vi "tvac_gui.vi"() -> ()   [LabVIEW 2017]
uses:
  <vilib>/httpClient/ClientHandle.ctl
  msg7171_linux.llb/send single message.vi
  <vilib>/httpClient/POSTBuffer.vi
  <vilib>/httpClient/LabVIEWHTTPClient.lvlib
panel:
  in  "Local Debug":bool
  out "Index Values":u32[](array[numeric])
  in  "NumberTCs":i32=120
  in  "Tab Control":enum32{"TCs"}(tab)
  in  "Graphing Selection":u16(ring) items=["User Selection", "Graph All Thermocouples", "Clear Graph"]
  in  "Time Scale":u16(ring) items=["Minutes", "Hours", "Seconds"]
  out "Waveform Chart":waveform(dbl)[](graph)
  out "Thermocouples":T1(array[cluster])
  in  "exit":bool
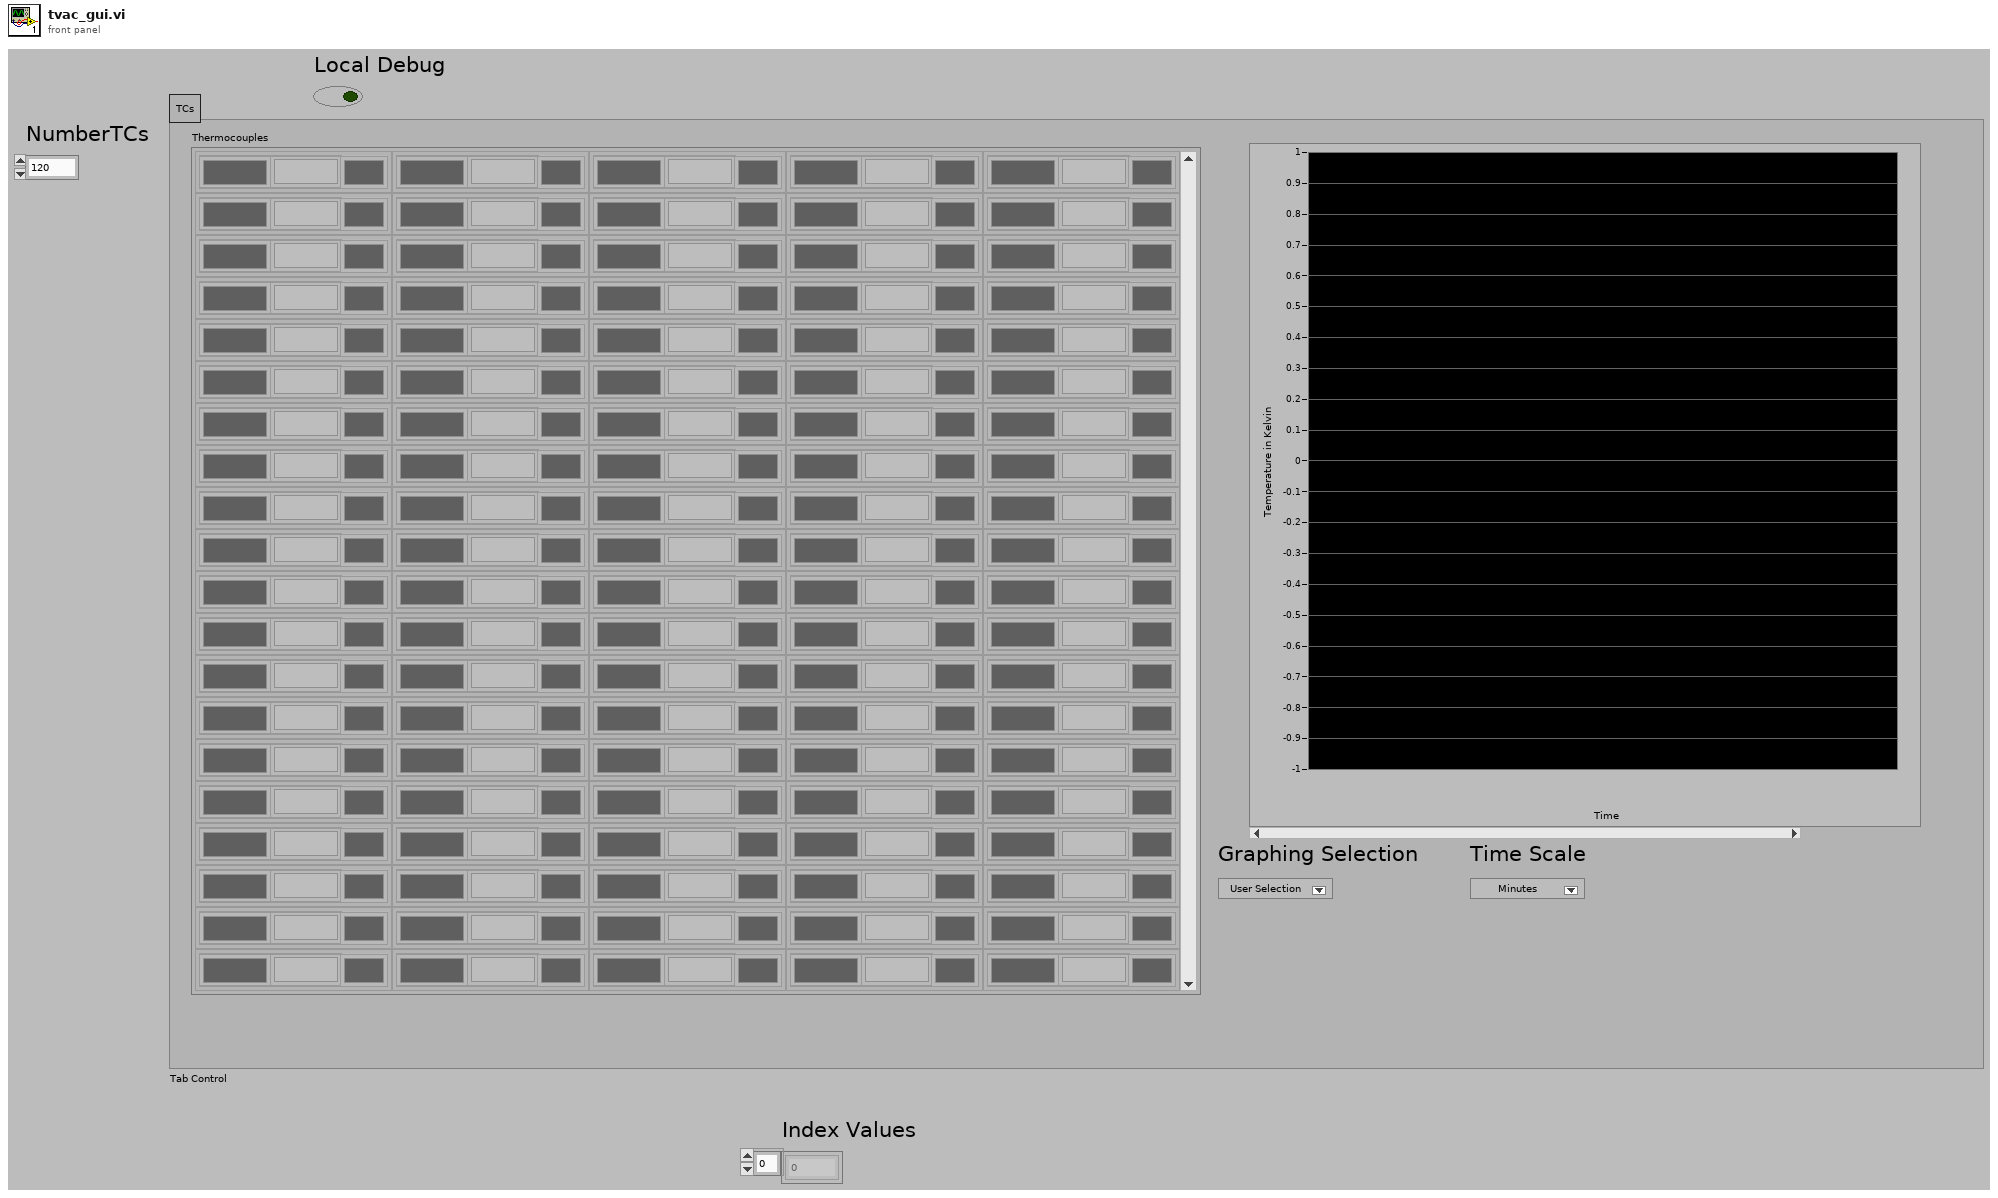
[diagram p1: front panel]
types:
  T1 = cluster{"TC Label":string, "Alarm Status":string, "Alarm Color":u32, "Temperature":string, "PlotColor":u32, "Graph On/Off":u32}[][]
  T2 = typedef "LabVIEWHTTPClient.lvlib/ClientHandle.ctl" = refnum<k1>
  T3 = cluster{"go":bool, "Http session":T2, "URL prefex":string}
  T4 = typedef "LVPoint32TypeDef.ctl" = cluster{"Horizontal":i32, "Vertical":i32}
  T5 = typedef "LVPositionTypeDef.ctl" = cluster{"Left":i32, "Top":i32}
  T6 = cluster{"TC Label":string, "Alarm Status":string, "Alarm Color":u32, "Temperature":string, "PlotColor":u32, "Graph On/Off":u32}
  T7 = typedef "LVRangeTypeDef.ctl" = cluster{"Minimum":dbl, "Maximum":dbl, "Increment":dbl, "Minor Increment":dbl, "Start":dbl}
  T8 = cluster{"time":string, "TCs":cluster{"thermocouple":i32, "time":dbl, "temp":dbl, "working":bool, "alarm":i32}[]}
  T9 = cluster{"thermocouple":i32, "time":dbl, "temp":dbl, "working":bool, "alarm":i32}[]
  T10 = cluster{"thermocouple":i32, "time":dbl, "temp":dbl, "working":bool, "alarm":i32}
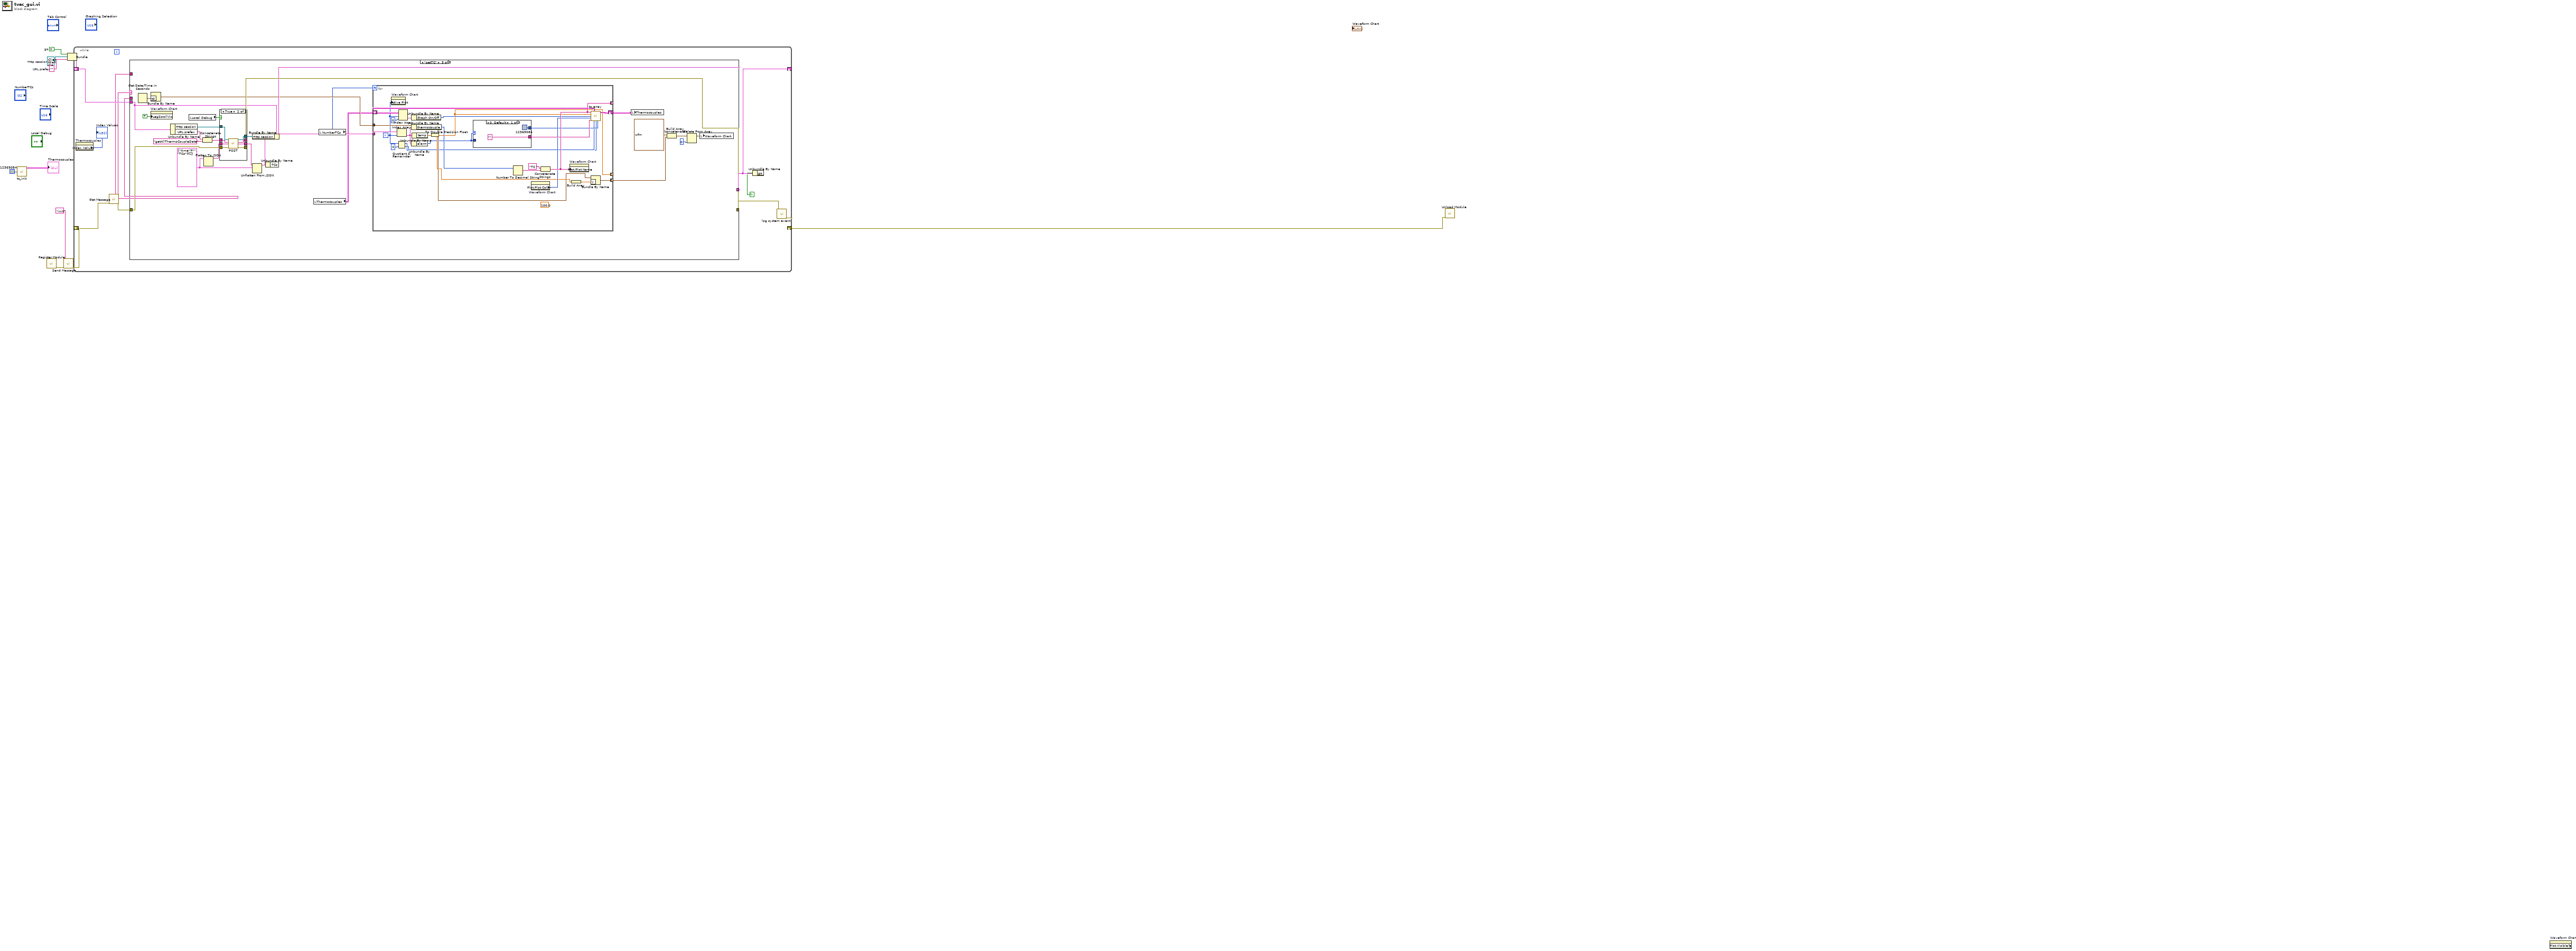
[diagram p0: block diagram]
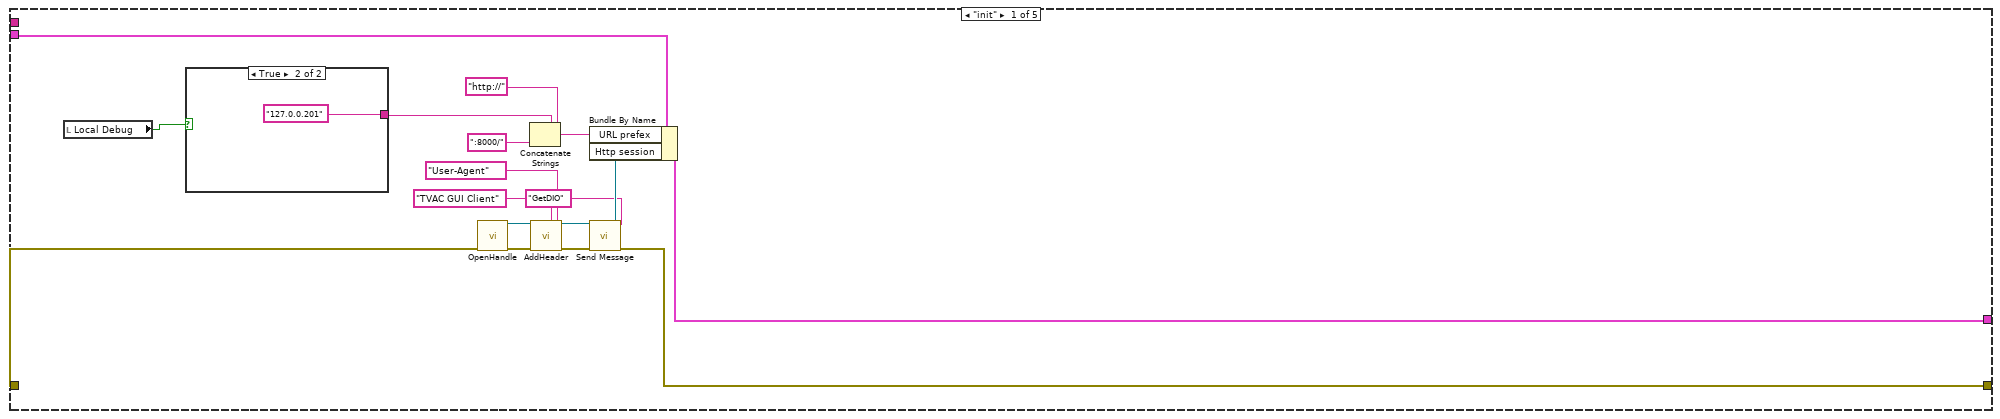
[diagram p2: hidden frame]
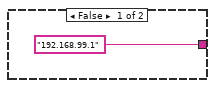
[diagram p3: hidden frame]
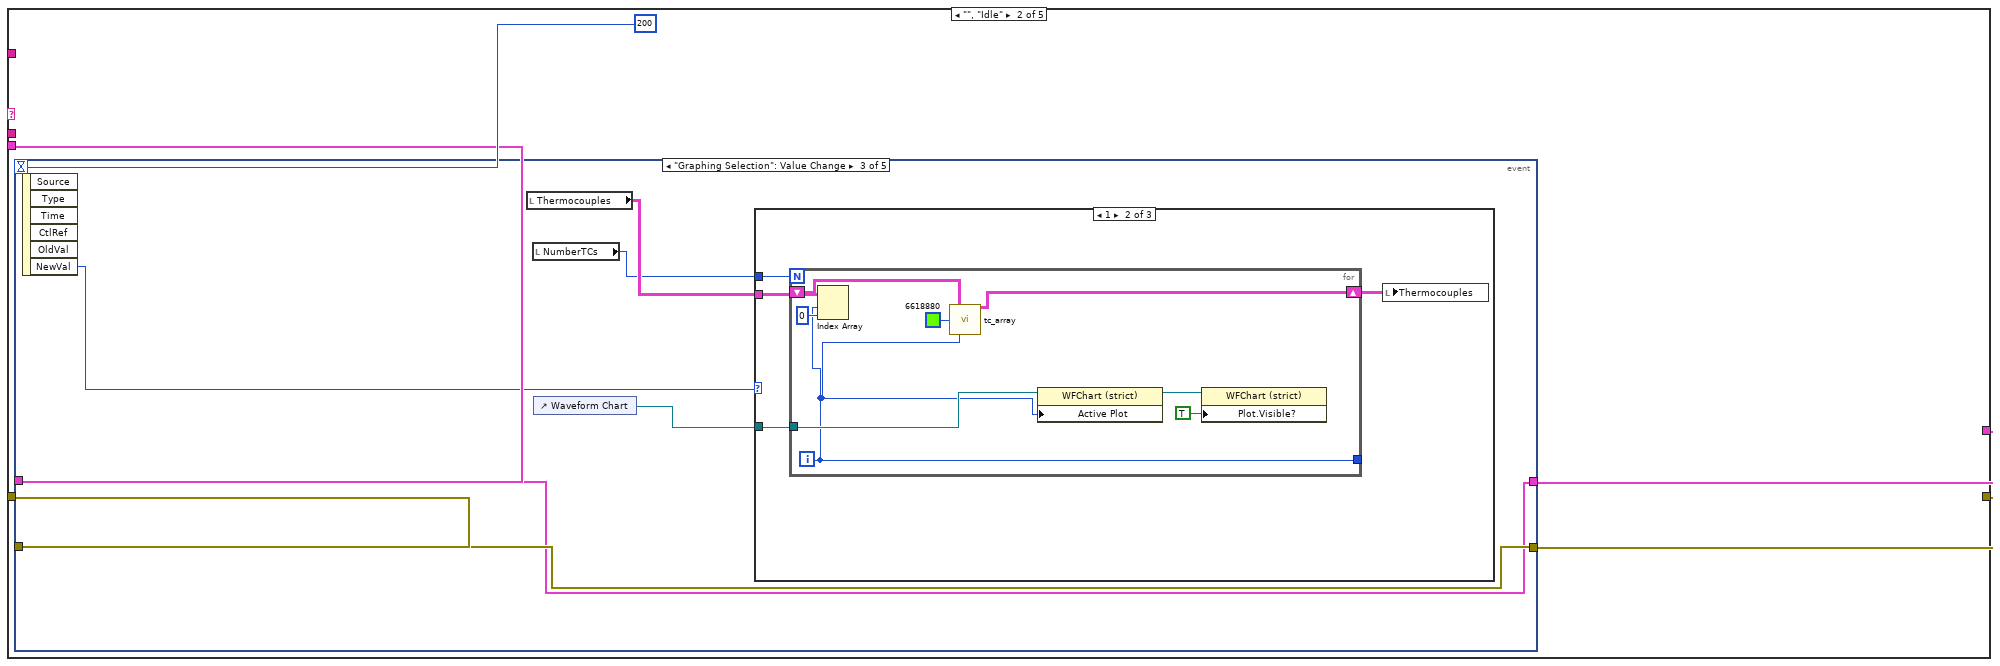
[diagram p4: hidden frame]
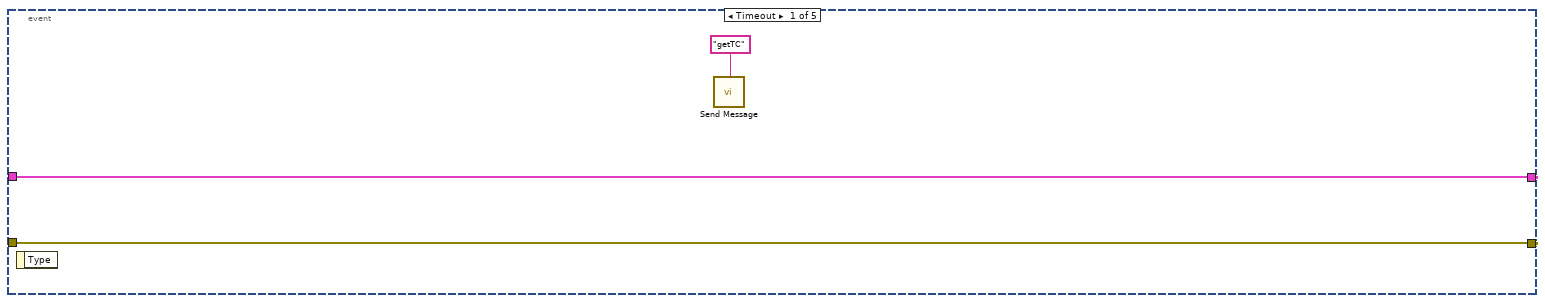
[diagram p5: hidden frame]
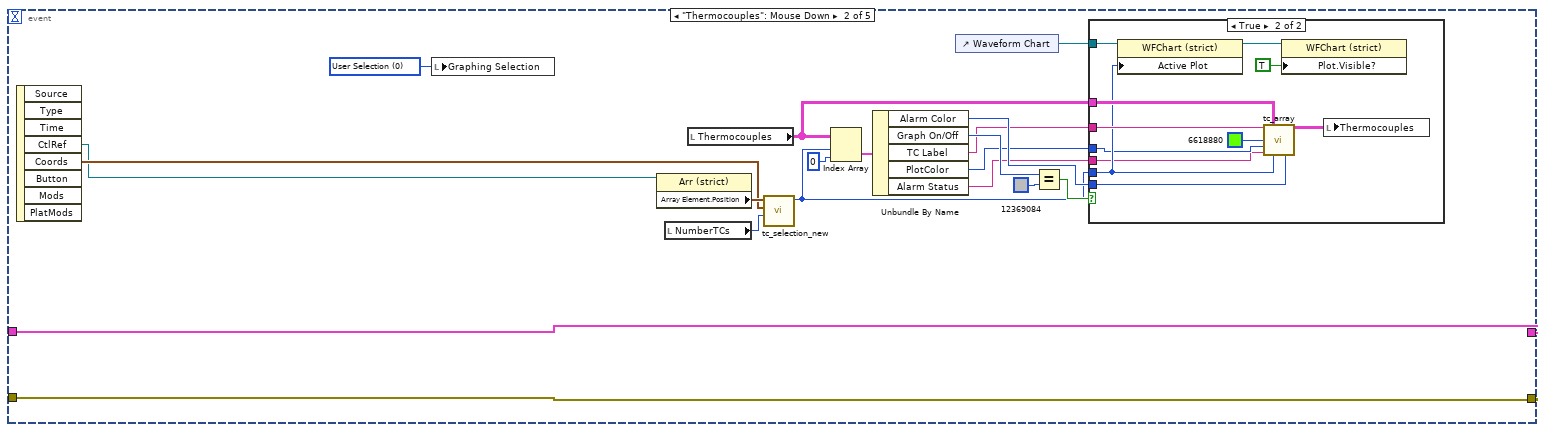
[diagram p6: hidden frame]
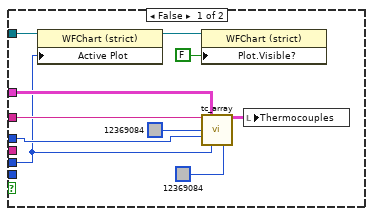
[diagram p7: hidden frame]
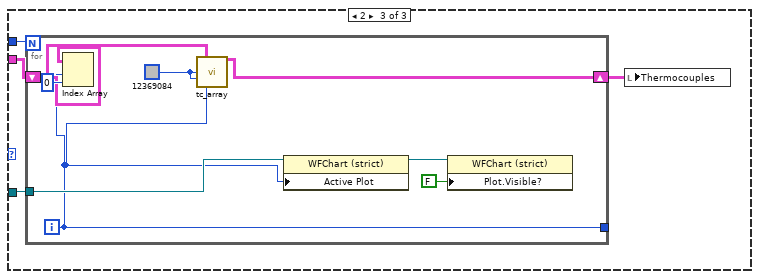
[diagram p9: hidden frame]
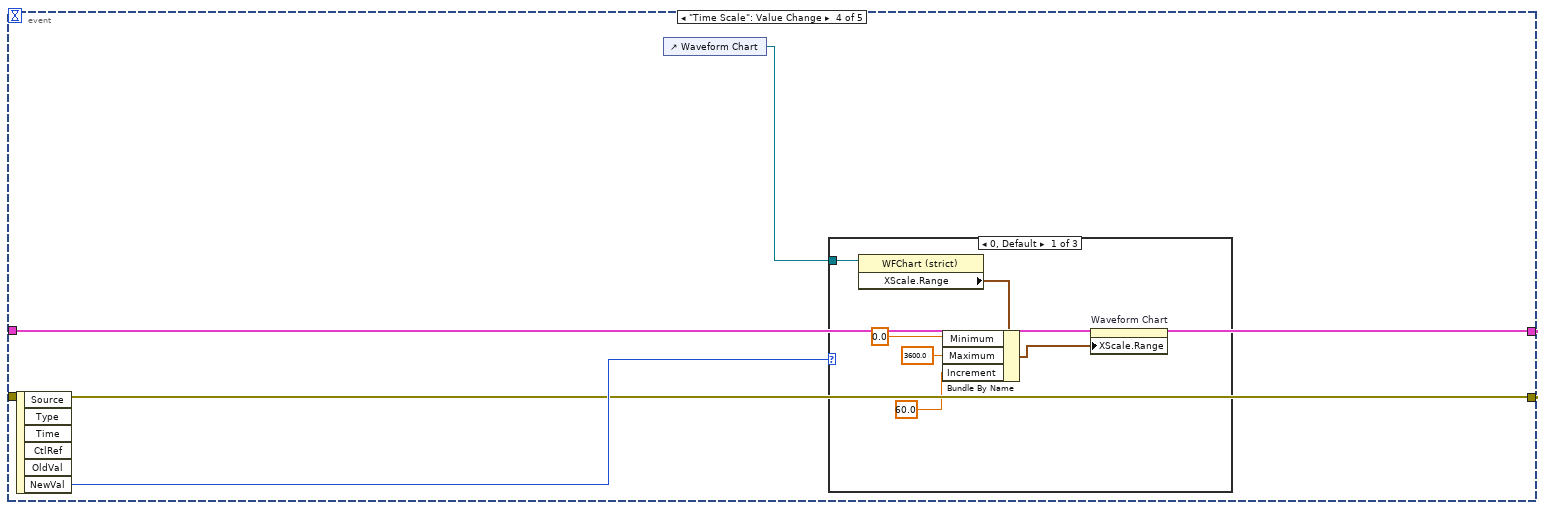
[diagram p10: hidden frame]
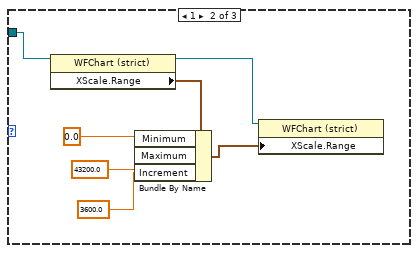
[diagram p11: hidden frame]
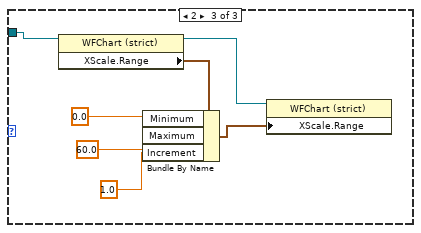
[diagram p12: hidden frame]
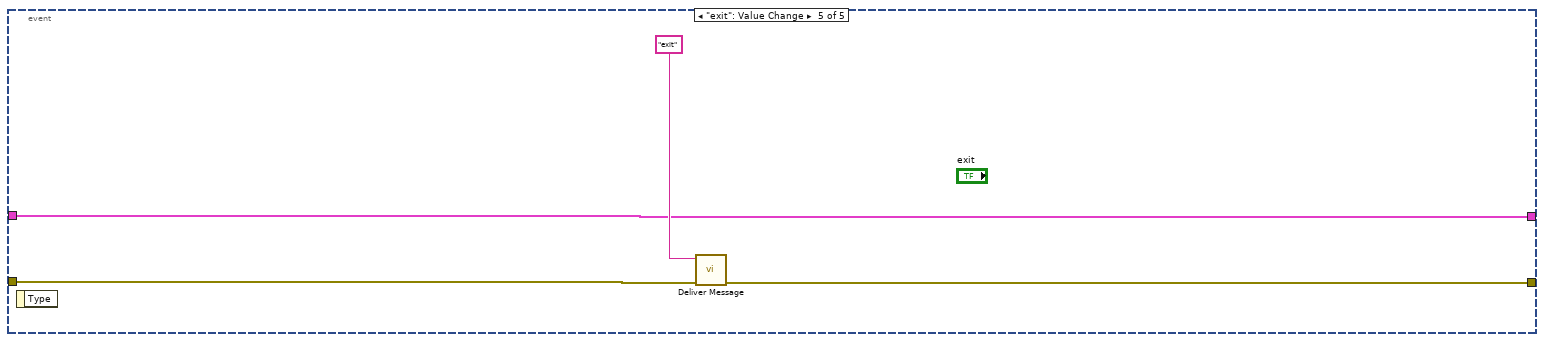
[diagram p13: hidden frame]
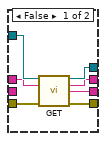
[diagram p14: hidden frame]
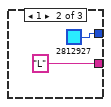
[diagram p15: hidden frame]
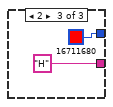
[diagram p16: hidden frame]
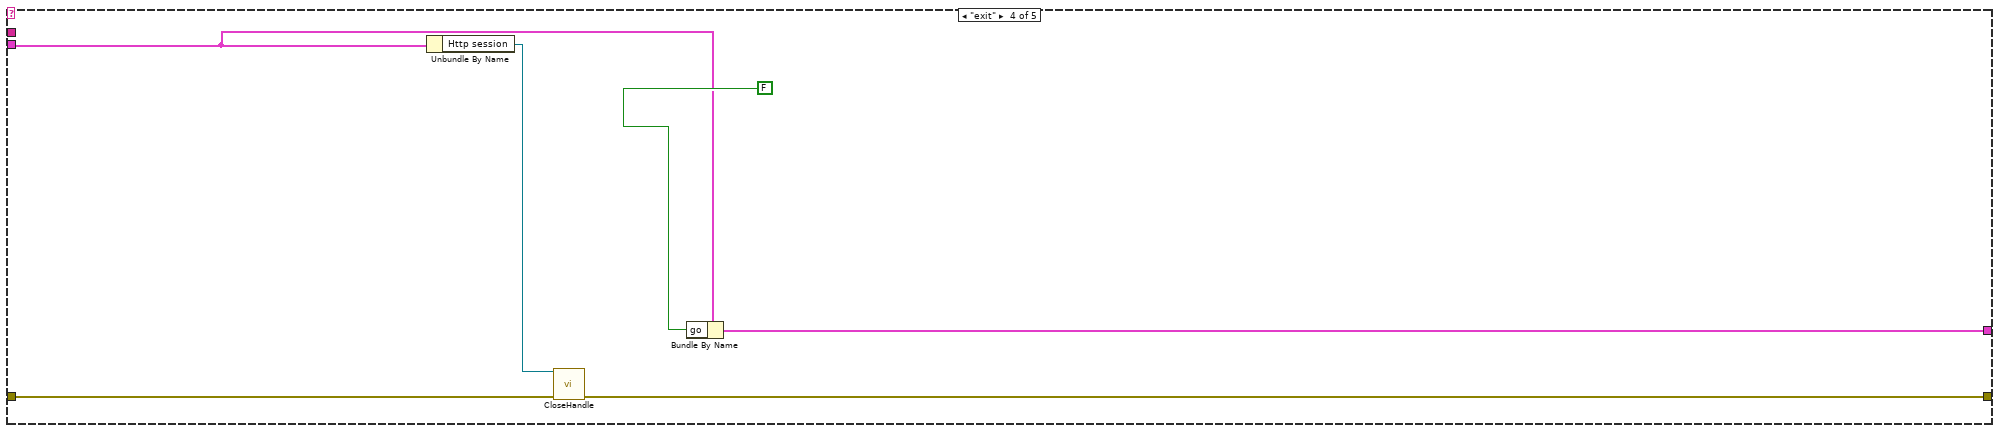
[diagram p17: hidden frame]
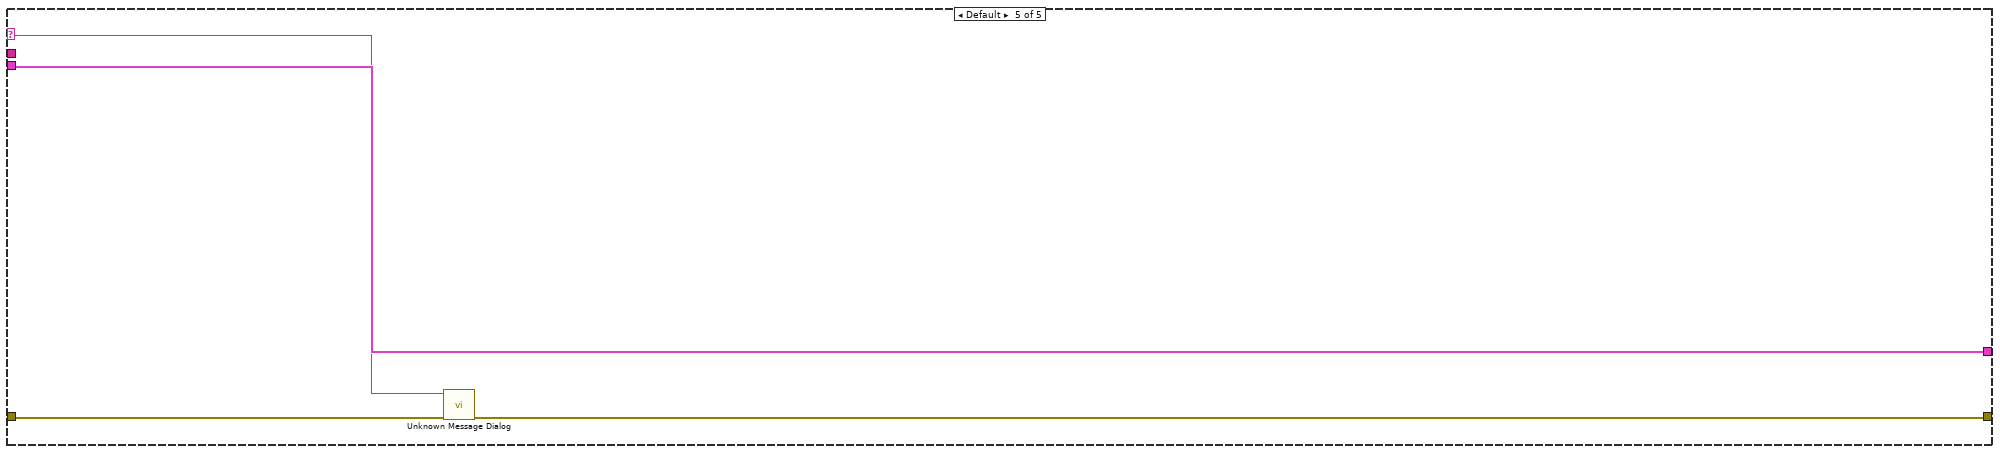
[diagram p18: hidden frame]
diagram:
  w6 = ""  # URL prefex
  w7 = T2 refnum  # Http session
  w8 = TRUE  # go
  n1 = call "tc_init.vi"("Graph ON/OFF"=u32 12369084) -> ("output array"=→"Thermocouples":T1)  [unwired: 14 in]
  n2 = call "Register Module.vi"() -> ("error out"=w4:errorcluster)  [unwired: 10 in, 1 out]
  n3 = call-poly "Send Message.vi"("error in (no error)"=w4, "event"="init") -> ("error out"=w3:errorcluster)  [unwired: 9 in]
  n4 = Bundle("go"=w8, "Http session"=w7, "URL prefex"=w6) -> (w10:T3)  [unwired: 1 in]
  n5 = while {
    shift-left: w10 -> [w18]
    shift-right: [w16] -> _
    shift-right: [w15] -> w9
    shift-left: w3 -> [w21]
    stop <- w12 continue-if-true
    n6 = property on="Thermocouples" class="Arr (strict)"() -> ("Index Values"=→"Index Values":u32[])  [unwired: 2 in, 2 out]
    n7 = call "Get Message.vi"("error in (no error)"=w21) -> ("error out"=w19:errorcluster, "event buffer"=w20:string, "event"=w17:string, "source"=w13:string)  [unwired: 7 in]
    n8 = case shown="\"getTC\"" w17 {
      selector: w17 -> [_ _ _ _ w224]
      tunnel: [w29 w41 w169 w222 w226] -> w16
      tunnel: w18 -> [w37 w40 w167 w217 w226]
      tunnel: w20 -> [_ _ _ _ _]
      tunnel: w19 -> [w32 w42 w171 w220 w225]
      tunnel: [w25 w44 w170 w219 w223] -> w14
      tunnel: w13 -> [_ _ _ _ _]
      frame "init" {
        n9 = local read "Local Debug"() -> (w22:bool)
        n10 = case shown="True" w22 {
          tunnel: ["192.168.99.1" ("Address") "127.0.0.201" ("Address")] -> w23
          frame False {
          }
          frame True {
          }
        }
        n11 = call <vilib>:"OpenHandle.vi"("error in (no error)"=w32) -> ("client handle out"=w33:T2, "error out"=w36:errorcluster)  [unwired: 13 in]
        n12 = Concatenate Strings("http://" ("url"), w23, ":8000/" ("url")) -> (w28:string)
        n13 = call <vilib>:"AddHeader.vi"("client handle"=w33, "header"="User-Agent", "value"="TVAC GUI Client", "error in (no error)"=w36) -> ("client handle out"=w27:T2, "error out"=w26:errorcluster)  [unwired: 10 in]
        n14 = Bundle By Name(cluster=w37, "URL prefex"=w28, "Http session"=w27) -> (w29:T3)
        n15 = call-poly "Send Message.vi"("error in (no error)"=w26, "event"="GetDIO") -> ("error out"=w25:errorcluster)  [unwired: 9 in]
      }
      frame "", "Idle" {
        n16 = event shown="[2] \"Graphing Selection\": Value Change" {
          selector: _ -> [_ _ _ _ _]
          dyn-events: _ -> [_ _ _ _ _]
          timeout: 200 ("milliseconds to wait") -> [_ _ _ _ _]
          tunnel: w42 -> [w46 w66 w89 w119 w145]
          tunnel: [w46 w66 w89 w119 w144] -> w44
          tunnel: [w47 w65 w88 w120 w142] -> w41
          tunnel: w40 -> [w47 w65 w88 w120 w142]
          event Timeout {
            n17 = event-data() -> ()  [unwired: 1 in, 1 out]
            n18 = call-poly "Send Message.vi"("event"="getTC") -> ()  [unwired: 10 in, 1 out]
          }
          event "Thermocouples": Mouse Down {
            w48 = u16 0 items=["User Selection", "Graph All Thermocouples", "Clear Graph"] ("Graphing Selection")
            n19 = event-data() -> ("CtlRef"=w62:refnum<vi>, "Coords"=w63:T4)  [unwired: 1 in, 6 out]
            n20 = local write "Graphing Selection"(w48) -> ()
            n21 = property class="Arr (strict)"(reference=w62) -> ("Array Element.Position"=w64:T5)  [unwired: 1 in, 2 out]
            n22 = local read "NumberTCs"() -> (w54:i32)
            n23 = local read "Thermocouples"() -> (w56:T1)
            n24 = call "tc_selection_new.vi"("Numeric 2"=w54, "Coords"=w63, "Position"=w64) -> ("Numeric"=w50:i32)  [unwired: 8 in]
            n25 = Index Array(array=w56, index (row)=w50, index (col)=0 ("disabled index (col)")) -> (element=w59:T6)
            n26 = Unbundle By Name(w59) -> ("Alarm Color"=w55:u32, "Graph On/Off"=w53:u32, "TC Label"=w52:string, "PlotColor"=w51:u32, "Alarm Status"=w49:string)
            n27 = control-ref of="Waveform Chart"() -> (w57:refnum<vi>)
            n28 = Equal?(x=w53, y=u32 12369084) -> (x = y?=w58:bool)
            n29 = case shown="True" w58 {
              tunnel: w50 -> [w68 w80]
              tunnel: w57 -> [w74 w85]
              tunnel: w56 -> [w70 w82]
              tunnel: w55 -> [_ w77]
              tunnel: w52 -> [w72 w84]
              tunnel: w51 -> [w69 w79]
              tunnel: w49 -> [_ w78]
              frame False {
                n30 = property on="Property Node" class="WFChart (strict)"(reference=w74, "Active Plot"=w68) -> (reference out=w75:refnum<vi>)  [unwired: 1 in, 1 out]
                n31 = property class="WFChart (strict)"(reference=w75, "Plot.Visible?"=FALSE ("Plot.Visible")) -> ()  [unwired: 1 in, 2 out]
                n32 = call "tc_array.vi"("TC Label"=w72, "output array 2"=w70, "Graph ON/OFF"=u32 12369084, "Plot Color"=w69, "index (row)"=w68, "AlarmColor"=u32 12369084) -> ("output array"=w71:T1)  [unwired: 9 in]
                n33 = local write "Thermocouples"(w71) -> ()
              }
              frame True {
                n34 = property class="WFChart (strict)"(reference=w85, "Active Plot"=w80) -> (reference out=w86:refnum<vi>)  [unwired: 1 in, 1 out]
                n35 = call "tc_array.vi"("TC Label"=w84, "output array 2"=w82, "Graph ON/OFF"=u32 6618880, "Plot Color"=w79, "Alarm String"=w78, "index (row)"=w80, "AlarmColor"=w77) -> ("output array"=w81:T1)  [unwired: 8 in]
                n36 = property class="WFChart (strict)"(reference=w86, "Plot.Visible?"=TRUE ("Plot.Visible")) -> ()  [unwired: 1 in, 2 out]
                n37 = local write "Thermocouples"(w81) -> ()
              }
            }
          }
          event "Graphing Selection": Value Change {
            n38 = event-data() -> ("NewVal"=w90:u16)  [unwired: 1 in, 5 out]
            n39 = local read "Thermocouples"() -> (w93:T1)
            n40 = local read "NumberTCs"() -> (w91:i32)
            n41 = control-ref of="Waveform Chart"() -> (w92:refnum<vi>)
            n42 = case shown="1" w90 {
              tunnel: w93 -> [_ w97 w108]
              tunnel: w92 -> [_ w96 w107]
              tunnel: w91 -> [_ w95 w109]
              frame 0, Default {
              }
              frame 1 {
                n43 = for {
                  N: w95 -> [_]
                  tunnel: w96 -> [w102]
                  tunnel: [w101] -> _
                  shift-right: [w99] -> w94
                  shift-left: w97 -> [w100]
                  i -> [w101]
                  n44 = Index Array(array=w100, index (row)=w101, index (col)=0 ("disabled index (col)")) -> ()  [unwired: 1 out]
                  n45 = call "tc_array.vi"("output array 2"=w100, "Graph ON/OFF"=u32 6618880, "index (row)"=w101) -> ("output array"=w99:T1)  [unwired: 12 in]
                  n46 = property class="WFChart (strict)"(reference=w102, "Active Plot"=w101) -> (reference out=w104:refnum<vi>)  [unwired: 1 in, 1 out]
                  n47 = property class="WFChart (strict)"(reference=w104, "Plot.Visible?"=TRUE ("Plot.Visible")) -> ()  [unwired: 1 in, 2 out]
                }
                n48 = local write "Thermocouples"(w94) -> ()
              }
              frame 2 {
                n49 = for {
                  N: w109 -> [_]
                  tunnel: w107 -> [w114]
                  tunnel: [w112] -> _
                  shift-right: [w110] -> w106
                  shift-left: w108 -> [w113]
                  i -> [w112]
                  w111 = u32 12369084
                  n50 = Index Array(array=w113, index (row)=w112, index (col)=0 ("disabled index (col)")) -> ()  [unwired: 1 out]
                  n51 = call "tc_array.vi"("output array 2"=w113, "Graph ON/OFF"=w111, "Plot Color"=w111, "index (row)"=w112) -> ("output array"=w110:T1)  [unwired: 11 in]
                  n52 = property class="WFChart (strict)"(reference=w114, "Active Plot"=w112) -> (reference out=w116:refnum<vi>)  [unwired: 1 in, 1 out]
                  n53 = property class="WFChart (strict)"(reference=w116, "Plot.Visible?"=FALSE ("Plot.Visible")) -> ()  [unwired: 1 in, 2 out]
                }
                n54 = local write "Thermocouples"(w106) -> ()
              }
            }
          }
          event "Time Scale": Value Change {
            n55 = event-data() -> ("NewVal"=w121:u16)  [unwired: 1 in, 5 out]
            n56 = control-ref of="Waveform Chart"() -> (w118:refnum<vi>)
            n57 = case shown="0, Default" w121 {
              tunnel: w118 -> [w125 w129 w136]
              frame 0, Default {
                n58 = property on="Property Node" class="WFChart (strict)"(reference=w125) -> ("XScale.Range"=w127:T7)  [unwired: 1 in, 2 out]
                n59 = Bundle By Name(cluster=w127, "Minimum"=0.0, "Maximum"=3600.0, "Increment"=60.0) -> (w126:T7)
                n60 = property on="Waveform Chart" class="WFChart (strict)"("XScale.Range"=w126) -> ()  [unwired: 2 in, 2 out]
              }
              frame 1 {
                n61 = property on="Property Node" class="WFChart (strict)"(reference=w129) -> (reference out=w128:refnum<vi>, "XScale.Range"=w134:T7)  [unwired: 1 in, 1 out]
                n62 = Bundle By Name(cluster=w134, "Minimum"=0.0, "Maximum"=43200.0, "Increment"=3600.0) -> (w130:T7)
                n63 = property on="Property Node" class="WFChart (strict)"(reference=w128, "XScale.Range"=w130) -> ()  [unwired: 1 in, 2 out]
              }
              frame 2 {
                n64 = property on="Property Node" class="WFChart (strict)"(reference=w136) -> (reference out=w135:refnum<vi>, "XScale.Range"=w141:T7)  [unwired: 1 in, 1 out]
                n65 = Bundle By Name(cluster=w141, "Minimum"=0.0, "Maximum"=60.0, "Increment"=1.0) -> (w137:T7)
                n66 = property on="Property Node" class="WFChart (strict)"(reference=w135, "XScale.Range"=w137) -> ()  [unwired: 1 in, 2 out]
              }
            }
          }
          event "exit": Value Change {
            n67 = event-data() -> ()  [unwired: 1 in, 1 out]
            n68 = call "Deliver Message.vi"("error in (no error)"=w145, "event"="exit") -> ("error out"=w144:errorcluster)  [unwired: 9 in]
          }
        }
      }
      frame "getTC" {
        w148 = T8 {"time"="", "TCs"=[]} ("Cluster")
        n69 = Get Date/Time In Seconds() -> (seconds since 1Jan1904=w157:timestamp)
        n70 = Bundle By Name("t0"=w157) -> (w156:waveform(dbl))  [unwired: 1 in]
        n71 = property on="Waveform Chart" class="WFChart (strict)"("LegScrollVis"=TRUE ("Legend:Scrollbar Visible")) -> ()  [unwired: 2 in, 2 out]
        n72 = Unbundle By Name(w167) -> ("Http session"=w166:T2, "URL prefex"=w164:string)
        n73 = local read "Local Debug"() -> (w146:bool)
        n74 = Concatenate Strings(w164, "getAllThermoCoupleData" ("url")) -> (w165:string)
        n75 = Flatten To JSON(anything=w148) -> (JSON string=w147:string)  [unwired: 2 in, 1 out]
        n76 = case shown="True" w146 {
          tunnel: w171 -> [w178 w179]
          tunnel: [w177 w180] -> w170
          tunnel: [w176 w181] -> w168
          tunnel: w166 -> [w175 w184]
          tunnel: w165 -> [w174 w185]
          tunnel: [w173 w182] -> w162
          tunnel: [w172 w183] -> _
          tunnel: w147 -> [_ w186]
          frame False {
            n77 = call <vilib>:"GET.vi"("client handle"=w175, "url"=w174, "error in (no error)"=w178) -> ("client handle out"=w176:T2, "headers"=w172:string, "body"=w173:string, "error out"=w177:errorcluster)  [unwired: 9 in]
          }
          frame True {
            n78 = call-poly <vilib>:"POST.vi"("client handle"=w184, "url"=w185, "buffer"=w186, "error in (no error)"=w179) -> ("client handle out"=w181:T2, "headers"=w183:string, "body"=w182:string, "error out"=w180:errorcluster)  [unwired: 8 in]
          }
        }
        n79 = Bundle By Name(cluster=w167, "Http session"=w168) -> (w169:T3)
        n80 = Unflatten From JSON(JSON string=w162, type and defaults=w148) -> (value=w161:T8)  [unwired: 5 in, 1 out]
        n81 = Unbundle By Name(w161) -> ("TCs"=w160:T9)
        n82 = local read "Thermocouples"() -> (w152:T1)
        n83 = local read "NumberTCs"() -> (w149:i32)
        n84 = for {
          N: w149 -> [_]
          tunnel: w160 -> [w210]
          tunnel: w156 -> [w208]
          tunnel: [w209] -> w155 mode=indexing
          tunnel: [w192] -> _ mode=indexing
          tunnel: [w198] -> _ mode=indexing
          shift-right: [w199] -> w153
          shift-left: w152 -> [w197]
          i -> [w189]
          (unwired) 100.0 ("x")
          n85 = property on="Waveform Chart" class="WFChart (strict)"("Active Plot"=w189) -> ()  [unwired: 2 in, 2 out]
          n86 = Quotient & Remainder(x=w189, y=4) -> (x-y*floor(x/y)=w187:i32, floor(x/y)=w188:i32)
          n87 = Index Array(array=w210, index=w189) -> (element=w202:T10)
          n88 = Index Array(array=w197, index (row)=w189, index (col)=0 ("disabled index (col)")) -> (element=w201:T6)
          n89 = Unbundle By Name(w201) -> ("Graph On/Off"=w194:u32)
          n90 = Unbundle By Name(w202) -> ("thermocouple"=w206:i32)
          n91 = Unbundle By Name(w202) -> ("alarm"=w191:i32)
          n92 = Unbundle By Name(w202) -> ("temp"=w204:dbl)
          n93 = To Double Precision Float(number=w204) -> (double precision float=w192:dbl)
          n94 = case shown="0, Default" w191 {
            tunnel: ["" "L" "H"] -> w196
            tunnel: w191 -> [_ _ _]
            tunnel: [u32 12369084 u32 2812927 u32 16711680] -> w193
            frame 0, Default {
            }
            frame 1 {
            }
            frame 2 {
            }
          }
          n95 = Number To Decimal String(number=w206) -> (decimal integer string=w207:string)  [unwired: 1 in]
          n96 = property on="Waveform Chart" class="WFChart (strict)"() -> ("Plot.Plot Color"=w195:u32)  [unwired: 2 in, 2 out]
          n97 = Concatenate Strings("TC " ("string"), w207) -> (w198:string)
          n98 = property on="Waveform Chart" class="WFChart (strict)"("Plot.Plot Name"=w198) -> ()  [unwired: 2 in, 2 out]
          n99 = Build Array(w192) -> (w203:dbl[])
          n100 = call "tc_array.vi"("TC Label"=w198, "output array 2"=w197, "Temperature"=w192, "Graph ON/OFF"=w194, "Plot Color"=w195, "Alarm String"=w196, "index (row)"=w188, "index (col)"=w187, "AlarmColor"=w193) -> ("output array"=w199:T1)  [unwired: 6 in]
          n101 = Bundle By Name(cluster=w208, "Y"=w203) -> (w209:waveform(dbl))
        }
        n102 = local write "Thermocouples"(w153) -> ()
        n103 = Build Array (concatenate)(waveform(dbl) {"t0"=timestamp(0 s since 1904-01-01), "dt"=1.0, "Y"=[]} ("element"), w155) -> (w159:waveform(dbl)[])
        n104 = Delete From Array(array=w159, index=0) -> (array with subset deleted=w150:waveform(dbl)[])  [unwired: 1 in, 1 out]
        n105 = local write "Waveform Chart"(w150) -> ()
      }
      frame "exit" {
        n106 = Unbundle By Name(w217) -> ("Http session"=w218:T2)
        n107 = call <vilib>:"CloseHandle.vi"("client handle"=w218, "error in (no error)"=w220) -> ("error out"=w219:errorcluster)  [unwired: 13 in]
        n108 = Bundle By Name(cluster=w217, "go"=FALSE ("Bundle Element")) -> (w222:T3)
      }
      frame Default {
        n109 = call "Unknown Message Dialog.vi"("error in (no error)"=w225, "event name"=w224) -> ("error out"=w223:errorcluster)  [unwired: 9 in]
      }
    }
    n110 = Unbundle By Name(w16) -> ("go"=w12:bool)
    n111 = call "log system event.vi"("error in (no error)"=w14) -> ("error out"=w15:errorcluster)  [unwired: 9 in, 1 out]
  }
  n112 = call "Unload Module.vi"("error in (no error)"=w9) -> ()  [unwired: 10 in, 1 out]
  n113 = property on="Waveform Chart" class="WFChart (strict)" props=["Plot", "Visible?"]() -> ()  [unwired: 2 in, 3 out]
